vi "Output Bool To Byte.vi"(11 "Output Settings":bool[](array[boolean])) -> (3 "Output Settings out":u8[](array[numeric]) format="%.0x")   [LabVIEW 2018, in "PIOD.lvlib" / "PIOD.lvclass"]
uses:
  PIOD.lvclass
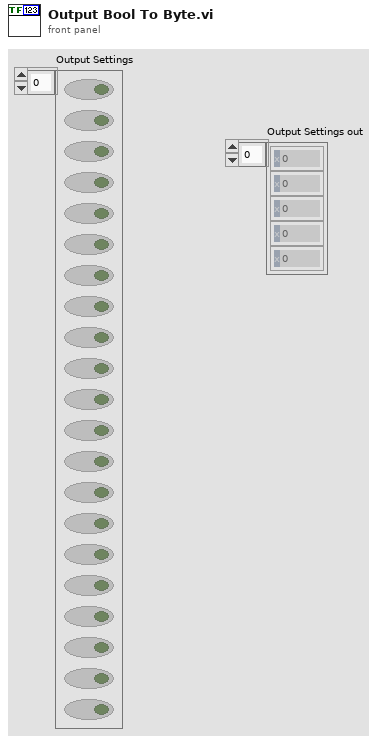
[diagram p1: front panel]
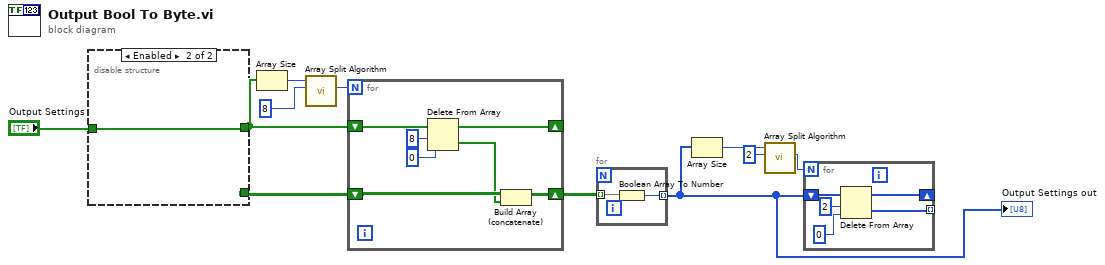
[diagram p0: block diagram]
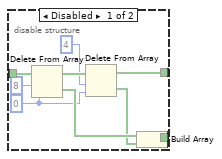
[diagram p2: hidden frame]
diagram:
  n1 = disable-structure shown="Enabled" {
    disable-tunnel: [w16 w21] -> w11
    disable-tunnel: [w15 _] -> w10
    disable-tunnel: "Output Settings" -> [w12 w21]
    frame Disabled {
      w13 = 0 ("index")
      n2 = Delete From Array(array=w12, length=8, index=w13) -> (deleted portion=w18:bool[], array with subset deleted=w19:bool[])
      n3 = Delete From Array(array=w19, length=4, index=w13) -> (deleted portion=w17:bool[], array with subset deleted=w16:bool[])
      n4 = Build Array(w18, w17) -> (w15:bool[][])
    }
    frame Enabled {
    }
  }
  n5 = Array Size(array=w11) -> (size(s)=w8:i32)
  n6 = call "Array Split Algorithm.vi"("Modulus"=8 ("y"), "Array Size"=w8) -> ("Loop counter"=w6:i32)  [unwired: 9 in]
  n7 = for {
    N: w6 -> [_]
    shift-right: [w25] -> _
    shift-left: w11 -> [w26]
    shift-right: [w23] -> w9
    shift-left: w10 -> [w24]
    n8 = Delete From Array(array=w26, length=8, index=0) -> (deleted portion=w22:bool[], array with subset deleted=w25:bool[])
    n9 = Build Array (concatenate)(w24, w22) -> (w23:bool[][])
  }
  n10 = for {
    tunnel: w9 -> [w30] mode=indexing
    tunnel: [w29] -> w2 mode=indexing
    n11 = Boolean Array To Number(Boolean array=w30) -> (number=w29:u8)
  }
  "Output Settings out" <- w2
  n12 = Array Size(array=w2) -> (size(s)=w5:i32)
  n13 = call "Array Split Algorithm.vi"("Modulus"=2, "Array Size"=w5) -> ("Loop counter"=w3:i32)  [unwired: 9 in]
  n14 = for {
    N: w3 -> [_]
    tunnel: [w34] -> _ mode=indexing
    shift-right: [w31] -> _
    shift-left: w2 -> [w35]
    n15 = Delete From Array(array=w35, length=2, index=0) -> (deleted portion=w34:u8[], array with subset deleted=w31:u8[])
  }
